vi "Action Stop.vi"(5 "Retry Attempts (0)":i32 min=0, 7 "Unit Address (-1)":i32=-1, 8 "error in (no error)":errorcluster, 11 "VISA resource name (in)":refnum<visa-resource-name>) -> (0 "error out":errorcluster, 2 "Response Cluster":T1 {"Command ID" format="%x"}, 3 "VISA resource name (out)":refnum<visa-resource-name>)   [LabVIEW 2020, in "Omega Platinum Series.lvlib"]
doc: "Sets the system state of the controller to STOP."
uses:
  Omega Platinum Series.lvlib
  Type Defs/Response.ctl
  Type Defs/System State.ctl
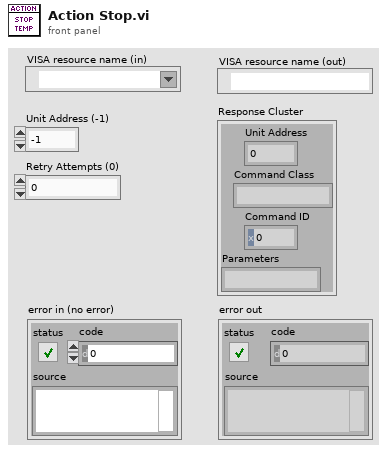
[diagram p1: front panel]
types:
  T1 = typedef "Omega Platinum Series.lvlib/Response.ctl" = cluster{"Unit Address":i32, "Command Class":string, "Command ID":u32, "Parameters":string}
  T2 = typedef "Omega Platinum Series.lvlib/System State.ctl" = enum16{"LOAD", "IDLE", "INPUT_ADJUST", "CONTROL_ADJUST", "MODIFY", "WAIT", "RUN", "STANDBY", "STOP", "PAUSE", "FAULT", "SHUTDOWN", "AUTOTUNE"}
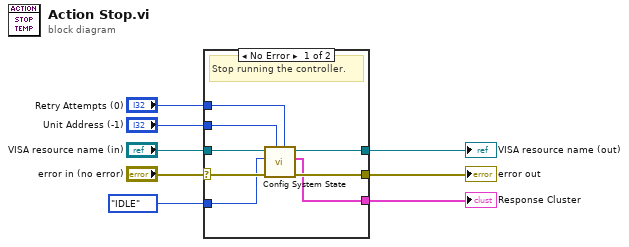
[diagram p0: block diagram]
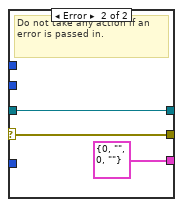
[diagram p2: hidden frame]
diagram:
  n1 = case shown="No Error" "error in (no error)" {
    selector: "error in (no error)" -> [w14 w19]
    tunnel: "Unit Address (-1)" -> [w12 _]
    tunnel: [w13 w19] -> w6
    tunnel: "VISA resource name (in)" -> [w16 w18]
    tunnel: [w15 w18] -> w4
    tunnel: [w10 T1 {"Unit Address"=0, "Command Class"="", "Command ID"=0, "Parameters"=""} ("Response Cluster")] -> w3
    tunnel: System_State."IDLE" ("System State") -> [w11 _]
    tunnel: "Retry Attempts (0)" -> [w9 _]
    frame No Error {
      # "Stop running the controller."
      n2 = call "Config System State.vi"("Retry Attempts (0)"=w9, "Unit Address (-1)"=w12, "error in (no error)"=w14, "System State"=w11, "VISA resource name (in)"=w16) -> ("error out"=w13:errorcluster, "Response Cluster"=w10:T1, "VISA resource name (out)"=w15:refnum<visa-resource-name>)  [unwired: 4 in]
    }
    frame Error {
      # "Do not take any action if an error is passed in."
    }
  }
  "error out" <- w6
  "VISA resource name (out)" <- w4
  "Response Cluster" <- w3
